vi "Stop Core.vi"(10 "final error code":i32, 11 "Game State in":refnum<class "Game State.lvclass">) -> (3 "Game State out":refnum<class "Game State.lvclass">)   [LabVIEW 2021, in "Game State Actor.lvlib" / "Game State.lvclass"]
uses:
  Game State.lvclass
  <vilib>/ActorFramework/Time-Delayed Send Message/Time-Delay Override Options.ctl
  Game State.lvclass/Game State.ctl
  <vilib>/ActorFramework/Actor/Actor.lvclass
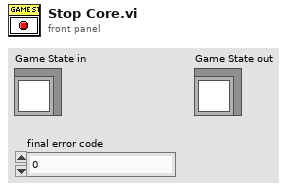
[diagram p1: front panel]
types:
  T1 = typedef "Time-Delay Override Options.ctl" = enum16{"Send next copy now", "Skip next scheduled copy", "Send next copy now and stop all further copies", "Stop all further copies"}
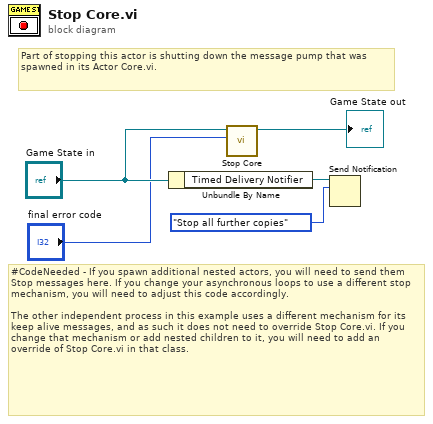
[diagram p0: block diagram]
diagram:
  # "#CodeNeeded - If you spawn additional nested actors, you will need to send them Stop messages here. If you change your asynchronous loops to use a different stop mechanism, you will need to adjust this code accordingly.\n\nThe other independent process in this example uses a different mechanism for its keep alive messages, and as such it does not need to override Stop Core.vi. If you change that mechanism or add nested children to it, you will need to add an override of Stop Core.vi in that class."
  # "Part of stopping this actor is shutting down the message pump that was spawned in its Actor Core.vi."
  n1 = Unbundle By Name("Game State in") -> ("Timed Delivery Notifier"=w3:refnum<notifier>)
  n2 = call-parent "Stop Core.vi"("final error code"="final error code", "Actor in"="Game State in") -> ("Actor out"=→"Game State out":refnum<class "Game State.lvclass">)  [unwired: 9 in]
  n3 = Send Notification(notification=Time-Delay_Override_Options."Stop all further copies", notifier=w3) -> ()  [unwired: 1 in, 2 out]
